vi "test-linear-filter-test-00.vi"() -> ()   [LabVIEW 2019]
uses:
  <vilib>/Rock Robotics/WPI/ThirdParty/JAS_Junk/TrajLib/Trajectory_Library.lvlib
panel:
  out "Output":dbl format="%13.5p"
  in  "Input":dbl format="%13.5p"
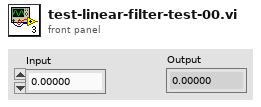
[diagram p1: front panel]
types:
  T1 = enum16{"Moving Average", "Low Pass 1st Order Butterworth", "Low Pass 2nd Order Butterworth", "High Pass 1st Order Butterworth", "High Pass 2nd Order Butterworth"}
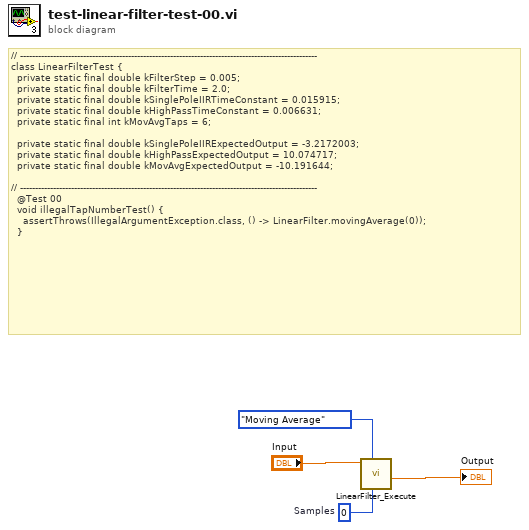
[diagram p0: block diagram]
diagram:
  w4 = 0  # Samples
  # "// ---------------------------------------------------------------------------------------------------\nclass LinearFilterTest {\n  private static final double kFilterStep = 0.005;\n  private static final double kFilterTime = 2.0;\n  private static final double kSinglePoleIIRTimeConstant = 0.015915;\n  private static final double kHighPassTimeConstant = 0.006631;\n  private static final int kMovAvgTaps = 6;\n\n  private static final double kSinglePoleIIRExpectedOutput = -3.2172003;\n  private static final double kHighPassExpectedOutput = 10.074717;\n  private static final double kMovAvgExpectedOutput = -10.191644;\n\n// ---------------------------------------------------------------------------------------------------\n  @Test 00\n  void illegalTapNumberTest() {\n    assertThrows(IllegalArgumentException.class, () -> LinearFilter.movingAverage(0));\n  }"
  n1 = call <vilib>:"LinearFilter_Execute.vi"("Samples"=w4, "Filter Type"=T1."Moving Average", "Input"="Input") -> ("Output"=→"Output":dbl)  [unwired: 7 in, 1 out]
